vi "Acquire Relative Reading.vi"(0 "VISA resource name":refnum<visa-resource-name>, 1 "Measurement (0: Voltage Channel 1)":i32(ring) items=["Voltage Channel 1", "Voltage Channel 2", "Temperature Channel 1", "Temperature Channel 2"], 11 "error in (no error)":errorcluster) -> (4 "VISA resource name out":refnum<visa-resource-name>, 15 "error out":errorcluster)   [LabVIEW 2019, in "Keithley 2182.lvlib"]
doc: "Acquires a reading to use as the reference (relative) value.\n\n<B>Note:</B>\nYou must first initialize a reading first. See <B>Keithley 2182 Relative Measurement</B> for example."
uses:
  Keithley 2182.lvlib
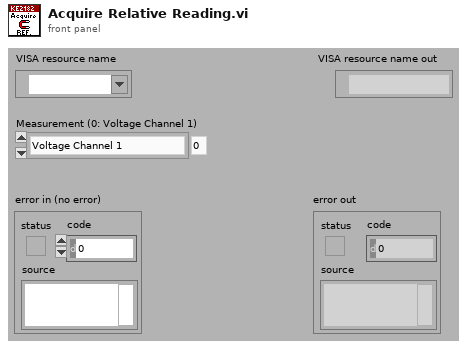
[diagram p1: front panel]
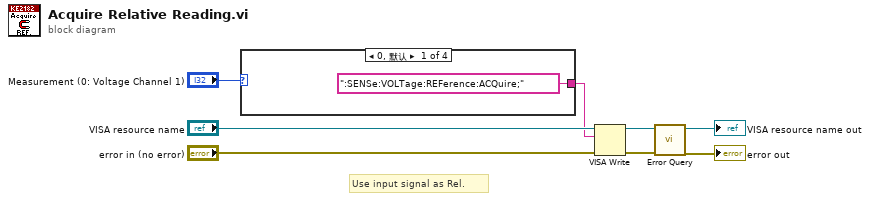
[diagram p0: block diagram]
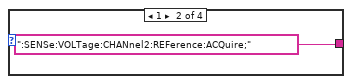
[diagram p2: hidden frame]
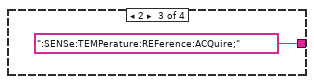
[diagram p3: hidden frame]
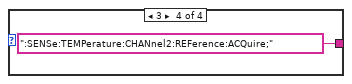
[diagram p4: hidden frame]
diagram:
  # "Use input signal as Rel."
  n1 = case shown="0, 默认" "Measurement (0: Voltage Channel 1)" {
    tunnel: [":SENSe:VOLTage:REFerence:ACQuire;" ":SENSe:VOLTage:CHANnel2:REFerence:ACQuire;" ":SENSe:TEMPerature:REFerence:ACQuire;" ":SENSe:TEMPerature:CHANnel2:REFerence:ACQuire;"] -> w1
    frame 0, Default {
    }
    frame 1 {
    }
    frame 2 {
    }
    frame 3 {
    }
  }
  n2 = VISA Write(VISA resource name="VISA resource name", write buffer=w1, error in (no error)="error in (no error)") -> (VISA resource name out=w6:refnum<visa-resource-name>, error out=w5:errorcluster)  [unwired: 1 out]
  n3 = call "Error Query.vi"("error in (no error)"=w5, "VISA resource name"=w6) -> ("error out"=→"error out":errorcluster, "VISA resource name out"=→"VISA resource name out":refnum<visa-resource-name>)  [unwired: 6 in, 2 out]
